vi "IPS120_GoToField.vi"(8 "error in":errorcluster, 11 "IPS120 Targets":T1={"Target Field (T)"=0.1, "Target Field Rate (T/min)"=0.1} {"Target Field (T)" format="%.4g"; "Target Field Rate (T/min)" format="%.4g"}) -> (0 "error out":errorcluster)   [LabVIEW 2016, in "IPS-120.lvlib" / "IPS-120-API.lvlib"]
doc: "Use this VI to remotely interact with the Oxford Mercury power supply through \"Oxford-1820-Main.vi\", which MUST also be running."
uses:
  IPS-120-API.lvlib
  Typedefs/Targets - Cluster.ctl
  IPS-120.lvlib
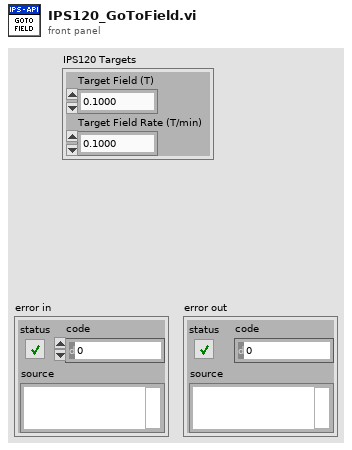
[diagram p1: front panel]
types:
  T1 = typedef "IPS-120.lvlib/Targets - Cluster.ctl" = cluster{"Target Field (T)":dbl, "Target Field Rate (T/min)":dbl}
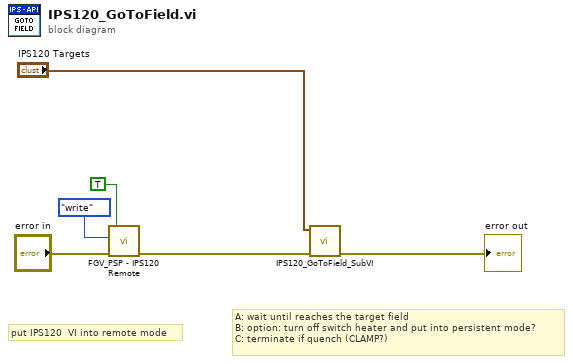
[diagram p0: block diagram]
diagram:
  # "A: wait until reaches the target field\nB: option: turn off switch heater and put into persistent mode?\nC: terminate if quench (CLAMP?)"
  # "put IPS120  VI into remote mode"
  n1 = call "FGV_PSP - IPS120 Remote.vi"("error in"="error in", "Function"=enum16{"write", "read"}."write", "Remote"=TRUE ("Mercury Remote")) -> ("error out"=w1:errorcluster)  [unwired: 3 in, 1 out]
  n2 = call "IPS120_GoToField_SubVI.vi"("error in (no error)"=w1, "Mercury Targets"="IPS120 Targets") -> ("error out"=→"error out":errorcluster)  [unwired: 9 in]
